vi "Error due to Cal Hole Distance.vi"(9 "Speed of Sound at Tc":dbl, 10 "Oscillator freq":i32, 11 "Cal Counts":i32) -> (2 "mm Error @ 10m":dbl, 3 "mm Error @ 5m":dbl)   [LabVIEW 2019, in "Analysis.lvlib"]
uses:
  Analysis.lvlib
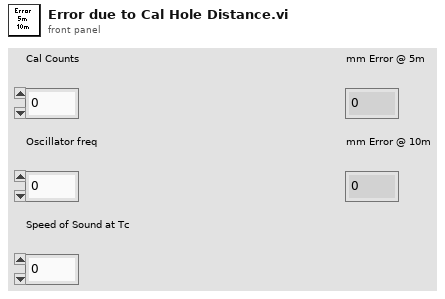
[diagram p1: front panel]
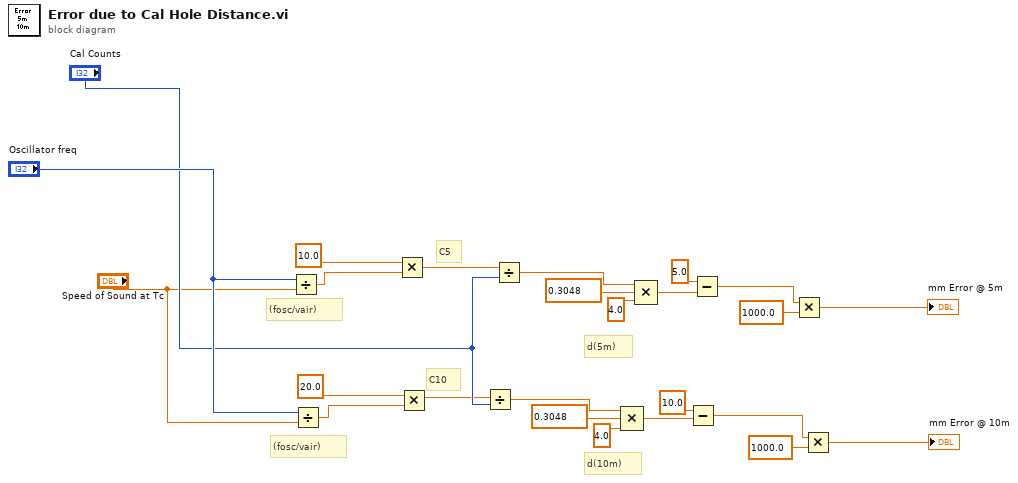
[diagram p0: block diagram]
diagram:
  # "(fosc/vair)"
  # "(fosc/vair)"
  # "C10"
  # "C5"
  # "d(10m)"
  # "d(5m)"
  n1 = Divide(x="Oscillator freq", y="Speed of Sound at Tc") -> (x/y=w13:dbl)
  n2 = Divide(x="Oscillator freq", y="Speed of Sound at Tc") -> (x/y=w14:dbl)
  n3 = Multiply(x=10.0 ("y"), y=w13) -> (x*y=w16:dbl)
  n4 = Multiply(x=20.0 ("y"), y=w14) -> (x*y=w17:dbl)
  n5 = Divide(x=w17, y="Cal Counts") -> (x/y=w12:dbl)
  n6 = Divide(x=w16, y="Cal Counts") -> (x/y=w8:dbl)
  n7 = Compound Arithmetic op=MULTIPLY(w12, 0.3048 ("y"), 4.0 ("y")) -> (w11:dbl)
  n8 = Compound Arithmetic op=MULTIPLY(w8, 0.3048 ("y"), 4.0 ("y")) -> (w7:dbl)
  n9 = Subtract(x=10.0 ("y"), y=w11) -> (x-y=w20:dbl)
  n10 = Subtract(x=5.0 ("y"), y=w7) -> (x-y=w23:dbl)
  n11 = Multiply(x=w23, y=1000.0) -> (x*y=→"mm Error @ 5m":dbl)
  n12 = Multiply(x=w20, y=1000.0) -> (x*y=→"mm Error @ 10m":dbl)
